vi "Get RC Config File Path.vi"(8 "Error In":errorcluster, 11 "Aircraft ID":u8) -> (0 "Error Out":errorcluster, 3 "Anchor Config File Path":path)   [LabVIEW 2014]
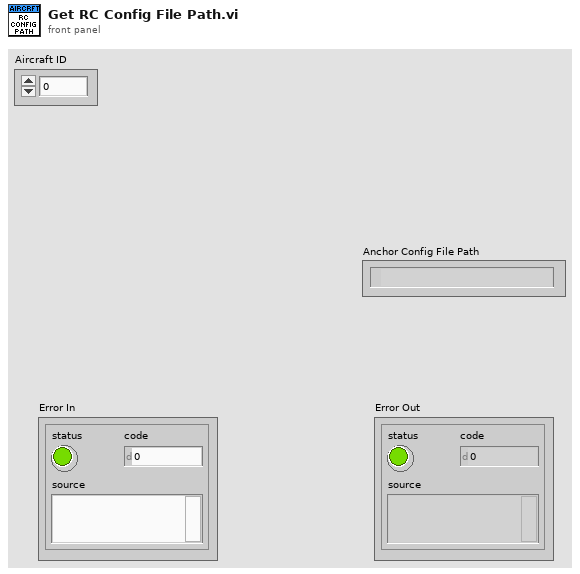
[diagram p1: front panel]
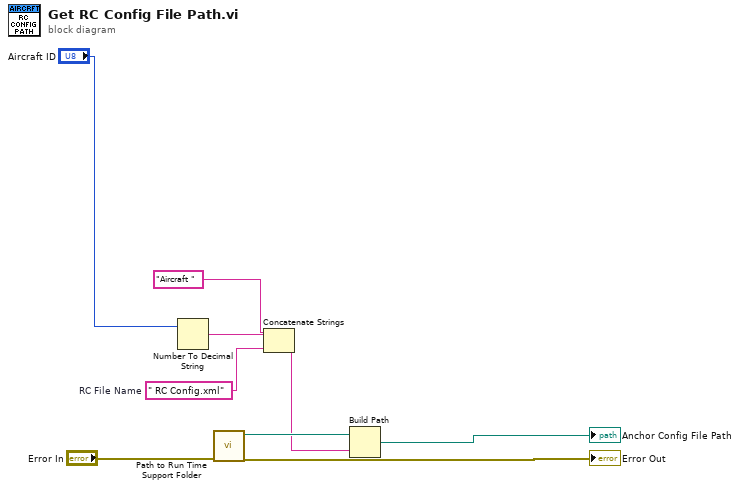
[diagram p0: block diagram]
diagram:
  w5 = " RC Config.xml"  # RC File Name
  n1 = Number To Decimal String(number="Aircraft ID") -> (decimal integer string=w2:string)  [unwired: 1 in]
  n2 = call "Path to Run Time Support Folder.vi"("Error In"="Error In") -> ("Error Out"=→"Error Out":errorcluster, "Path To Run Time Support Folder"=w9:path)  [unwired: 9 in]
  n3 = Concatenate Strings("Aircraft ", w2, w5) -> (w1:string)
  n4 = Build Path(base path=w9, name or relative path=w1) -> (appended path=→"Anchor Config File Path":path)
